vi "Start.vi"(7 "Targets":string[](array[string]), 8 "error in (no error)":errorcluster, 11 "Lock-In Remote Actor in":refnum<class "Lock-In Remote Actor.lvclass">) -> (0 "error out":errorcluster, 3 "Lock-In Remote Actor out":refnum<class "Lock-In Remote Actor.lvclass">)   [LabVIEW 2023, in "Lock-In Remote Actor.lvlib" / "Lock-In Remote Actor.lvclass"]
uses:
  Lock-In Remote Actor.lvclass
  Lock-In Remote Actor.lvclass/Lock-In Remote Actor.ctl
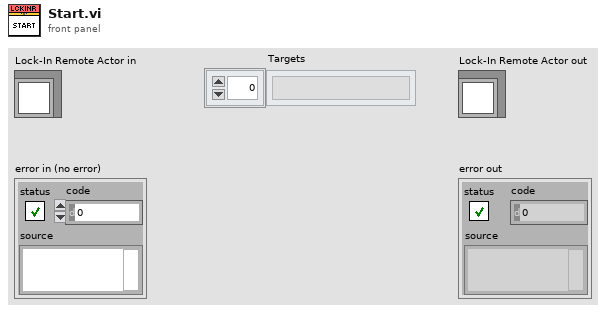
[diagram p1: front panel]
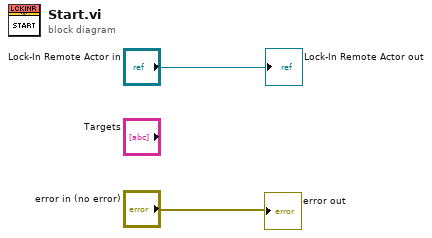
[diagram p0: block diagram]
diagram:
  "error out" <- "error in (no error)"
  "Lock-In Remote Actor out" <- "Lock-In Remote Actor in"
